vi "UHR-Fleezers Control (host) - 11.9c.vi"() -> ()   [LabVIEW 2014] (continued)
        n2850 = Multiply(x=w4184, y=u64 2) -> (x*y=w4169:u64)
        n2851 = call "integrate 1D array interval - double.vi"("Ave N"=w4186, "Array In"=w4185) -> ("Array Out"=w4197:dbl[])  [unwired: 1 out]
        n2852 = call "integrate 1D array interval - double.vi"("Ave N"=w4186, "Array In"=w4283) -> ("Array Out"=w4282:dbl[])  [unwired: 1 out]
        n2853 = Array Size(array=w4197) -> (size(s)=w4198:i32)
        n2854 = Array Size(array=w4282) -> (size(s)=w4284:i32)
        n2855 = Multiply(x=w4170, y=w4169) -> (x*y=w4200:u64)
        n2856 = Multiply(x=w4170, y=w4169) -> (x*y=w4292:u64)
        n2857 = call-poly <vilib>:"Mean.vi"("X"=w4232) -> ("mean"=w4216:dbl)  [unwired: 1 out]
        n2858 = Subtract(x=w4200, y=w4198) -> (x-y=w4191:u64)
        n2859 = call-poly <vilib>:"Mean.vi"("X"=w4234) -> ("mean"=w4221:dbl)  [unwired: 1 out]
        n2860 = call-poly <vilib>:"Mean.vi"("X"=w4233) -> ("mean"=w4219:dbl)  [unwired: 1 out]
        n2861 = call-poly <vilib>:"Mean.vi"("X"=w4197) -> ("mean"=w4188:dbl)  [unwired: 1 out]
        n2862 = Subtract(x=w4292, y=w4284) -> (x-y=w4226:u64)
        n2863 = call-poly <vilib>:"Mean.vi"("X"=w4282) -> ("mean"=w4223:dbl)  [unwired: 1 out]
        n2864 = Initialize Array(1.0 ("element"), w4191) -> (w4187:dbl[])
        n2865 = Initialize Array(1.0 ("element"), w4226) -> (w4217:dbl[])
        n2866 = Multiply(x=w4187, y=w4188) -> (x*y=w4189:dbl[])
        n2867 = Multiply(x=w4217, y=w4219) -> (x*y=w4220:dbl[])
        n2868 = Multiply(x=w4217, y=w4221) -> (x*y=w4222:dbl[])
        n2869 = Multiply(x=w4217, y=w4216) -> (x*y=w4218:dbl[])
        n2870 = Multiply(x=w4217, y=w4223) -> (x*y=w4224:dbl[])
        n2871 = Build Array (concatenate)(w4232, w4218) -> (w4286:dbl[])
        n2872 = Build Array (concatenate)(w4234, w4222) -> (w4290:dbl[])
        n2873 = Build Array (concatenate)(w4233, w4220) -> (w4289:dbl[])
        n2874 = Build Array (concatenate)(w4197, w4189) -> (w4199:dbl[])
        n2875 = Build Array (concatenate)(w4282, w4224) -> (w4291:dbl[])
        n2876 = Reshape Array(w4286, w4170, w4169) -> (w4252:dbl[][])
        n2877 = Reshape Array(w4199, w4170, w4169) -> (w4195:dbl[][])
        n2878 = Reshape Array(w4290, w4170, w4169) -> (w4244:dbl[][])
        n2879 = Reshape Array(w4289, w4170, w4169) -> (w4259:dbl[][])
        n2880 = Reshape Array(w4291, w4170, w4169) -> (w4269:dbl[][])
        n2881 = Array Subset(array=w4259, index (col)=0 ("index"), length (col)=w4184) -> (w4264:dbl[][])  [unwired: 2 in]
        n2882 = Array Subset(array=w4259, index (col)=w4184) -> (w4262:dbl[][])  [unwired: 3 in]
        n2883 = Array Subset(array=w4244, index (col)=0 ("index"), length (col)=w4184) -> (w4250:dbl[][])  [unwired: 2 in]
        n2884 = Array Subset(array=w4244, index (col)=w4184) -> (w4248:dbl[][])  [unwired: 3 in]
        n2885 = Array Subset(array=w4195, index (col)=0 ("index"), length (col)=w4184) -> (w4194:dbl[][])  [unwired: 2 in]
        n2886 = Array Subset(array=w4195, index (col)=w4184) -> (w4192:dbl[][])  [unwired: 3 in]
        n2887 = Array Subset(array=w4269, index (col)=0 ("index"), length (col)=w4184) -> (w4268:dbl[][])  [unwired: 2 in]
        n2888 = Array Subset(array=w4269, index (col)=w4184) -> (w4266:dbl[][])  [unwired: 3 in]
        n2889 = Array Subset(array=w4252, index (col)=0 ("index"), length (col)=w4184) -> (w4257:dbl[][])  [unwired: 2 in]
        n2890 = Array Subset(array=w4252, index (col)=w4184) -> (w4255:dbl[][])  [unwired: 3 in]
        n2891 = for {
          tunnel: w4264 -> [w4306] mode=indexing
          tunnel: [w4305] -> w4263 mode=indexing
          workers-P: _ -> [_]
          n2892 = Reverse 1D Array(array=w4306) -> (reversed array=w4305:dbl[])
        }
        n2893 = for {
          tunnel: w4250 -> [w4302] mode=indexing
          tunnel: [w4301] -> w4249 mode=indexing
          workers-P: _ -> [_]
          n2894 = Reverse 1D Array(array=w4302) -> (reversed array=w4301:dbl[])
        }
        n2895 = for {
          tunnel: w4194 -> [w4300] mode=indexing
          tunnel: [w4299] -> w4193 mode=indexing
          workers-P: _ -> [_]
          n2896 = Reverse 1D Array(array=w4300) -> (reversed array=w4299:dbl[])
        }
        n2897 = for {
          tunnel: w4268 -> [w4308] mode=indexing
          tunnel: [w4307] -> w4267 mode=indexing
          workers-P: _ -> [_]
          n2898 = Reverse 1D Array(array=w4308) -> (reversed array=w4307:dbl[])
        }
        n2899 = for {
          tunnel: w4257 -> [w4304] mode=indexing
          tunnel: [w4303] -> w4256 mode=indexing
          workers-P: _ -> [_]
          n2900 = Reverse 1D Array(array=w4304) -> (reversed array=w4303:dbl[])
        }
        n2901 = Index Array(array=w4269, index (row)=0) -> (element=→"Waveform Graph":dbl[])  [unwired: 1 in]
        n2902 = Add(x=w4263, y=w4262) -> (x+y=w4261:dbl[][])
        n2903 = Add(x=w4249, y=w4248) -> (x+y=w4247:dbl[][])
        n2904 = Add(x=w4193, y=w4192) -> (x+y=w4177:dbl[][])
        n2905 = Add(x=w4267, y=w4266) -> (x+y=w4241:dbl[][])
        n2906 = Add(x=w4256, y=w4255) -> (x+y=w4254:dbl[][])
        n2907 = Divide(x=w4247, y=2) -> (x/y=w4245:dbl[][])
        n2908 = Divide(x=w4261, y=2) -> (x/y=w4206:dbl[][])
        n2909 = Divide(x=w4254, y=2) -> (x/y=w4208:dbl[][])
        n2910 = To Single Precision Float(number=w4241) -> (single precision float=w4240:sgl[][])
        n2911 = Transpose 2D Array(2D array=w4245) -> (transposed array=→"Data map":dbl[][])
        n2912 = To Single Precision Float(number=w4177) -> (single precision float=w4181:sgl[][])
        n2913 = To Single Precision Float(number=w4206) -> (single precision float=w4212:sgl[][])
        n2914 = To Single Precision Float(number=w4208) -> (single precision float=w4209:sgl[][])
        n2915 = call "IMAQ ArrayToImage"("Image Pixels (Float)"=w4240, "Image"=w4174) -> ("Image Out"=w4243:T2)  [unwired: 8 in, 1 out]
        n2916 = call "IMAQ ArrayToImage"("Image Pixels (Float)"=w4181, "Image"=w4173) -> ("Image Out"=w4183:T2)  [unwired: 8 in, 1 out]
        n2917 = call "IMAQ ArrayToImage"("Image Pixels (Float)"=w4212, "Image"=w4172) -> ("Image Out"=w4214:T2)  [unwired: 8 in, 1 out]
        n2918 = call "IMAQ ArrayToImage"("Image Pixels (Float)"=w4209, "Image"=w4171) -> ("Image Out"=w4211:T2)  [unwired: 8 in, 1 out]
        n2919 = call "IMAQ Symmetry"("Type of Symmetry"=w4242, "Image Src"=w4243) -> ("Image Dst Out"=w4238:T2)  [unwired: 3 in, 1 out]
        n2920 = call "IMAQ Symmetry"("Type of Symmetry"=w4182, "Image Src"=w4183) -> ("Image Dst Out"=w4179:T2)  [unwired: 3 in, 1 out]
        n2921 = call "IMAQ Symmetry"("Type of Symmetry"=w4213, "Image Src"=w4214) -> ("Image Dst Out"=→"Detection Laser X":T2)  [unwired: 3 in, 1 out]
        n2922 = call "IMAQ Symmetry"("Type of Symmetry"=w4210, "Image Src"=w4211) -> ("Image Dst Out"=→"Detection Laser Y":T2)  [unwired: 3 in, 1 out]
        n2923 = call "IMAQ Set Simple Calibration"("Calibration Axis Info"=T37 {"Origin Pixel"={"X"=0.0, "Y"=0.0}, "Angle Relative to Horizontal (deg)"=0.0, "Axis Reference"=0}, "Grid Descriptor"=T38 {"X Step"=0.3, "Y Step"=0.3, "Unit"=enum."Undefined"}, "Image"=w4238) -> ("Calibrated Image"=→"APD 1":T2)  [unwired: 7 in, 1 out]
        n2924 = call "IMAQ Set Simple Calibration"("Calibration Axis Info"=T37 {"Origin Pixel"={"X"=0.0, "Y"=0.0}, "Angle Relative to Horizontal (deg)"=0.0, "Axis Reference"=0}, "Grid Descriptor"=T38 {"X Step"=0.3, "Y Step"=0.3, "Unit"=enum."Undefined"}, "Image"=w4179) -> ("Calibrated Image"=→"APD 2":T2)  [unwired: 7 in, 1 out]
      }
    }
    n2925 = Subtract(x=w3621, y="APD 2 Offset") -> (x-y=w3618:waveform(dbl))
    n2926 = Subtract(x=w3623, y="APD 1 Offset") -> (x-y=w3619:waveform(dbl))
    n2927 = Index Array(array=w3638, index=3) -> (element=w3698:waveform(dbl))
    n2928 = Index Array(array=w3638, index=6) -> (element=w3695:waveform(dbl))
    n2929 = Build Array(w3619, w3618) -> (→"APD Chart":waveform(dbl)[])
    n2930 = Array Size(array=w3689) -> (size(s)=w3742:i32)
    n2931 = call <vilib>:"Std Deviation and Variance.vi"("X"=w3631) -> ("standard deviation"=w3630:dbl)  [unwired: 1 in, 2 out]
    n2932 = Add Array Elements(numeric array=w3631) -> (sum=w3633:u32)
    n2933 = Add Array Elements(numeric array=w3689) -> (sum=w3752:u32)
    n2934 = call <vilib>:"Std Deviation and Variance.vi"("X"=w3689) -> ("standard deviation"=w3688:dbl)  [unwired: 1 in, 2 out]
    n2935 = Divide(x="T1 offset_x (mV)", y=1000.0) -> (x/y=w3699:dbl)
    n2936 = Divide(x=w3630, y=w3629) -> (x/y=w3626:dbl)
    "Rate sigma (Hz) 2" <- w3626
    n2937 = Multiply(x=w3629, y=w3742) -> (x*y=w3632:dbl)
    "Int. Time (s)" <- w3632
    n2938 = Divide(x=w3633, y=w3632) -> (x/y=w3627:dbl)
    "APD 2 Rate (Hz)" <- w3627
    n2939 = Divide(x=w3752, y=w3632) -> (x/y=w3686:dbl)
    "APD 1 Rate (Hz)" <- w3686
    n2940 = Divide(x=w3688, y=w3629) -> (x/y=w3687:dbl)
    "Rate sigma (Hz)" <- w3687
    n2941 = Divide(x=w3626, y=w3627) -> (x/y=→"Sigma/Mean 2":dbl)
    n2942 = Divide(x=w3687, y=w3686) -> (x/y=→"s/Mean":dbl)
    n2943 = feedback-in #26("Calibration") -> ()
    n2944 = feedback #26(u16 1 ("Calibration")) -> (w3719:u16)
    n2945 = Divide(x="T2 offset_x (mV)", y=1000.0) -> (x/y=w3697:dbl)
    n2946 = case shown="0, Default" "Calibration" {
      tunnel: "T1 a_x (nm/V)" -> [_ w4137 w4158]
      tunnel: "T1 k_x (pN/nm)" -> [_ _ w4148]
      tunnel: "T2 a_x (nm/V)" -> [_ w4136 w4156]
      tunnel: "T2 k_x (pN/nm)" -> [_ _ w4149]
      tunnel: w3698 -> [w4119 w4134 w4154]
      tunnel: w3695 -> [w4118 w4132 w4152]
      tunnel: [w4119 w4131 w4151] -> w3728
      tunnel: [w4118 w4130 w4150] -> w3727
      tunnel: ["T1 X (V)" ("Label.Text") "T1 X (nm)" ("Label.Text") "T1 X (pN)" ("Label.Text")] -> w3716
      tunnel: ["T2 X (V)" ("Label.Text") "T2 X (nm)" ("Label.Text") "T2 X (pN)" ("Label.Text")] -> w3715
      tunnel: ["Position (V)" ("Label.Text") "Position (nm)" ("Label.Text") "Force (pN)" ("Label.Text")] -> w3717
      tunnel: w3697 -> [_ w4122 w4141]
      tunnel: w3699 -> [_ w4125 w4143]
      tunnel: ["Mean (V)" ("Label.Text") "Mean (nm)" ("Label.Text") "Mean (pN)" ("Label.Text")] -> w3712
      tunnel: ["Difference (V)" ("Label.Text") "Difference (nm)" ("Label.Text") "Difference (pN)" ("Label.Text")] -> w3646
      frame 0, Default {
      }
      frame 1 {
        n2947 = Unbundle By Name(w4134) -> ("Y"=w4138:dbl[])
        n2948 = Unbundle By Name(w4132) -> ("Y"=w4123:dbl[])
        n2949 = Subtract(x=w4138, y=w4125) -> (x-y=w4126:dbl[])
        n2950 = Subtract(x=w4123, y=w4122) -> (x-y=w4124:dbl[])
        n2951 = Multiply(x=w4124, y=w4136) -> (x*y=w4133:dbl[])
        n2952 = Multiply(x=w4137, y=w4126) -> (x*y=w4135:dbl[])
        n2953 = Bundle By Name(cluster=w4132, "Y"=w4133) -> (w4130:waveform(dbl))
        n2954 = Bundle By Name(cluster=w4134, "Y"=w4135) -> (w4131:waveform(dbl))
      }
      frame 2 {
        n2955 = Unbundle By Name(w4154) -> ("Y"=w4159:dbl[])
        n2956 = Unbundle By Name(w4152) -> ("Y"=w4157:dbl[])
        n2957 = Subtract(x=w4157, y=w4141) -> (x-y=w4142:dbl[])
        n2958 = Subtract(x=w4159, y=w4143) -> (x-y=w4144:dbl[])
        n2959 = Compound Arithmetic op=MULTIPLY(w4142, w4156, w4149) -> (w4153:dbl[])
        n2960 = Compound Arithmetic op=MULTIPLY(w4148, w4158, w4144) -> (w4155:dbl[])
        n2961 = Bundle By Name(cluster=w4152, "Y"=w4153) -> (w4150:waveform(dbl))
        n2962 = Bundle By Name(cluster=w4154, "Y"=w4155) -> (w4151:waveform(dbl))
      }
    }
    n2963 = Not Equal?(x=w3719, y="Calibration") -> (x != y?=w3676:bool)
    n2964 = case shown="True" w3676 {
      tunnel: w3717 -> [_ w4112]
      tunnel: w3716 -> [_ w4111]
      tunnel: w3715 -> [_ w4110]
      tunnel: w3712 -> [_ w4109]
      tunnel: w3646 -> [_ w4108]
      frame False {
      }
      frame True {
        n2965 = property on="Force" class="WFChart (strict)"("YScale.NameLbl.Text"=w4112) -> ()  [unwired: 2 in, 2 out]
        n2966 = property on="T2 X" class="DigNum (strict)"("Caption.Text"=w4110) -> ()  [unwired: 2 in, 2 out]
        n2967 = property on="T1 X" class="DigNum (strict)"("Caption.Text"=w4111) -> ()  [unwired: 2 in, 2 out]
        n2968 = property on="Mean" class="DigNum (strict)"("Caption.Text"=w4109) -> ()  [unwired: 2 in, 2 out]
        n2969 = property on="Difference" class="DigNum (strict)"("Caption.Text"=w4108) -> ()  [unwired: 2 in, 2 out]
      }
    }
    n2970 = Unbundle By Name(w3698) -> ("Y"=w3701:dbl[])
    n2971 = Unbundle By Name(w3695) -> ("Y"=w3704:dbl[])
    n2972 = Subtract(x=w3701, y=w3699) -> (x-y=w3702:dbl[])
    n2973 = Subtract(x=w3704, y=w3697) -> (x-y=w3703:dbl[])
    n2974 = Multiply(x=w3703, y="T2 a_x (nm/V)") -> (x*y=w3491:dbl[])
    n2975 = Multiply(x="T1 a_x (nm/V)", y=w3702) -> (x*y=w3492:dbl[])
    n2976 = Not(x="Trap Trig. Fl.") -> (.not. x?=w3528:bool)
    n2977 = Multiply(x=w3727, y=-1.0) -> (x*y=w3706:waveform(dbl))
    n2978 = Subtract(x=w3492, y=w3491) -> (x-y=w3694:dbl[])
    n2979 = Unbundle By Name(w3727) -> ("Y"=w3665:dbl[])
    n2980 = Unbundle By Name(w3728) -> ("Y"=w3493:dbl[])
    n2981 = Negate(x=w3694) -> (-x=w3489:dbl[])
    n2982 = Build Array(w3728, w3706) -> (→"Force":waveform(dbl)[])
    n2983 = Subtract(x=w3489, y="Offset (nm)") -> (x-y=w3663:dbl[])
    n2984 = case shown="True" "Read Lateness and Rel Phase" {
      tunnel: w3509 -> [w4083 w4107]
      tunnel: w3508 -> [w4084 w4106]
      tunnel: [w4083 w4105] -> w3692
      tunnel: [w4084 w4104] -> w3691
      frame False {
      }
      frame True {
        n2985 = xnode "Read/Write Control"("FPGA VI Reference In"=w4107, "error in"=w4106) -> ("FPGA VI Reference Out"=w4105:T20, "error out"=w4104:errorcluster, "GI Relative phase"=→"GI relative phase":i16, "Relative phase"=→"Relative phase (AI1)":i16, "AI Late Counter"=→"Late Counter (AI1)":u8, "GI Late Counter"=→"GI Late Counter":u8, "MCL Late Counter"=→"MCL Late Counter":u8, "MCL Relative Phase"=→"Relative Phase (MCL)":i16, "APD Acq Relative Phase"=→"APD Acq Relative Phase":i16, "APD 1 Gate Relative Phase"=→"APD 1 Gate Relative Phase":i16, "APD 2 Gate Relative Phase"=→"APD 2 Gate Relative Phase":i16, "APD Acq Late Counter"=→"APD Acq Late Counter":u8, "APD 1 Gate Late Counter"=→"APD 1 Gate Late Counter":u8, "APD 2 Gate Late Counter"=→"APD 2 Gate Late Counter":u8, "Green FB Relative Phase"=→"Relative phase (Green FB)":i16, "GI Relative phase 2"=→"GI relative phase 2":i16, "GI Late Counter 2"=→"GI Late Counter 2":u8, "Trap Pos FIFO Timeout"=→"Trap Pos FIFO Timeout":u16, "Trap AI FIFO Timeout"=→"Trap AI FIFO Timeout":u16, "RI relative phase"=→"RI relative phase":i16, "RI late counter"=→"RI late counter":u8)
      }
    }
    n2986 = call-poly <vilib>:"Mean.vi"("X"=w3665) -> ("mean"=w3495:dbl)  [unwired: 1 out]
    "T2 X" <- w3495
    n2987 = Negate(x=w3665) -> (-x=w3666:dbl[])
    n2988 = call-poly <vilib>:"Mean.vi"("X"=w3493) -> ("mean"=w3496:dbl)  [unwired: 1 out]
    "T1 X" <- w3496
    n2989 = Negate(x=w3495) -> (-x=w3494:dbl)
    n2990 = Bundle By Name(cluster=w3698, "Y"=w3663) -> (w3637:waveform(dbl))
    "Bead Separation" <- w3637
    n2991 = Add(x=w3493, y=w3666) -> (x+y=w3667:dbl[])
    n2992 = Add(x=w3496, y=w3494) -> (x+y=w3714:dbl)
    n2993 = Subtract(x=w3496, y=w3494) -> (x-y=→"Difference":dbl)
    n2994 = Divide(x=w3667, y=2.0) -> (x/y=→"Vec Mean of T1 T2":dbl[])
    n2995 = Divide(x=w3714, y=2.0) -> (x/y=w3669:dbl)
    "Mean" <- w3669
    n2996 = feedback-in #27("Trap Trig. Fl.") -> ()
    n2997 = feedback #27("Trap Trig. Fl.") -> (w3526:bool)
    n2998 = And(x=w3528, y=w3526) -> (x .and. y?=w3527:bool)
    n2999 = case "If have just turned off triggering" shown="True" w3527 {
      tunnel: w3509 -> [_ w3913]
      tunnel: w3508 -> [_ w3912]
      frame False {
      }
      frame True {
        w3911 = FALSE ("FPGA Trap Trig")
        n3000 = xnode "Read/Write Control"("FPGA VI Reference In"=w3913, "error in"=w3912, "FPGA Trap Trig"=w3911) -> ("FPGA VI Reference Out"=w3910:T20, "error out"=w3909:errorcluster)
        n3001 = xnode "Read/Write Control"("FPGA VI Reference In"=w3910, "error in"=w3909, "TTrig?"=w3911) -> ()  [unwired: 2 out]
        n3002 = local write "Initializing"(FALSE ("Initializing")) -> ()
        n3003 = local write "Triggered"(FALSE ("Triggered")) -> ()
        n3004 = local write "Waiting"(FALSE ("Waiting")) -> ()
      }
    }
    n3005 = Not(x=w3526) -> (.not. x?=w3539:bool)
    n3006 = And(x="Trap Trig. Fl.", y=w3539) -> (x .and. y?=w3536:bool)
    n3007 = local read "Tether"() -> (w3670:bool)
    n3008 = Or(x=w3536, y="Reinitialize") -> (x .or. y?=w3522:bool)
    n3009 = feedback #28(w3532) -> (w3537:string)
    n3010 = Select(t=w3532, s=w3536, f=w3537) -> (s? t:f=w3531:string)
    n3011 = Select(t=w3532, s="Reinitialize", f=w3531) -> (s? t:f=w3530:string)
    n3012 = feedback #29(0) -> (w3534:i32)
    n3013 = feedback #30(w3663) -> (w3662:dbl[])
    n3014 = Build Array (concatenate)(w3663, w3662) -> (w3490:dbl[])
    n3015 = case "For determining if there is a tether still" shown="True" w3670 {
      tunnel: w3669 -> [_ w4037]
      frame False {
      }
      frame True {
        n3016 = Greater?(x="Lost Tether Alarm Threshold (pN)", y=w4037) -> (0:w4035:bool)
        n3017 = case shown="True" w4035 {
          frame False {
          }
          frame True {
            w4038 = TRUE
            w4042 = FALSE ("Multiple tether")
            w4043 = FALSE ("Value (Signaling)")
            n3018 = flat-sequence {
              frame #0 {
                # "stop only if saving"
                n3019 = local read "Saving..."() -> (w4055:bool)
                n3020 = And(x=w4055, y="TA Cancel Save?") -> (x .and. y?=w4054:bool)
                n3021 = local write "Stop Saving"(w4054) -> ()
              }
              frame #1 {
                n3022 = case shown="True" "TA Green Off?" {
                  frame False {
                  }
                  frame True {
                    w4058 = FALSE ("Fl. Triggered...")
                    n3023 = local write "Fl. Triggered..."(w4058) -> ()
                    n3024 = property on="Green ON/Interlacing" class="Bool (strict)"("Val(Sgnl)"=w4058) -> ()  [unwired: 2 in, 2 out]
                  }
                }
              }
            }
            n3025 = local read "Time tether formed"() -> (w4049:timestamp)
            n3026 = Get Date/Time In Seconds() -> (seconds since 1Jan1904=w4050:timestamp)
            n3027 = Subtract(x=w4050, y=w4049) -> (x-y=w4048:dbl)
            n3028 = Number To Decimal String(number=w4048) -> (decimal integer string=w4045:string)  [unwired: 1 out]
            n3029 = local read "Messages"() -> (w4052:string)
            n3030 = call <vilib>:"Beep.vi"("use system alert? (T)"=FALSE, "duration (msec)"=u32 200, "frequency (Hz)"=u32 200) -> ()  [unwired: 9 out]
            n3031 = Concatenate Strings("Lost tether (" ("Message to add"), w4045, " s)." ("string")) -> (w4047:string)
            n3032 = local write "Tether"(FALSE ("Tether")) -> ()
            n3033 = call "Update messages.vi"("Message to add"=w4047, "Old message string"=w4052) -> ("New message string"=w4051:string)
            n3034 = local write "Messages"(w4051) -> ()
            n3035 = local write "Pause dwell"(w4043) -> ()
            n3036 = property on="Fl. Triggered..." class="Bool (strict)"("Val(Sgnl)"=w4043) -> ()  [unwired: 2 in, 2 out]
            n3037 = local write "Dip for Protein"(w4043) -> ()
            n3038 = property on="Trap Pos. FB ON" class="Bool (strict)"("Val(Sgnl)"=w4043) -> ()  [unwired: 2 in, 2 out]
            n3039 = property on="Trap Trig. Fl." class="Bool (strict)"("Val(Sgnl)"=w4043) -> ()  [unwired: 2 in, 2 out]
            n3040 = local write "Multiple tether"(w4042) -> ()
            n3041 = local write "Bad fit"(w4042) -> ()
            n3042 = local write "Hysteresis"(w4042) -> ()
            n3043 = local write "Good tether"(w4042) -> ()
            n3044 = local write "Save scans"(w4038) -> ()
            n3045 = local write "Restart DMA? (AOD)"(w4038) -> ()
          }
        }
      }
    }
    n3046 = case "For triggering actions based on the trap position (e.g., turning the excitation laser on if trap under feedback moves so far)" shown="True" "Trap Trig. Fl." {
      tunnel: w3517 -> [_ w3926]
      tunnel: w3530 -> [_ w3925]
      tunnel: ["" ("t") w3924] -> w3538
      tunnel: w3522 -> [_ w3923]
      tunnel: [0 ("t") w3922] -> w3535
      tunnel: w3534 -> [_ w3921]
      tunnel: w3509 -> [_ w3920]
      tunnel: w3508 -> [_ w3919]
      frame False {
      }
      frame True {
        n3047 = case shown="\"Wait for trigger\"" w3925 {
          tunnel: w3926 -> [w3943 _ _ w3991]
          tunnel: [w3940 w3972 "" ("t") w3994] -> w3924
          tunnel: w3923 -> [_ _ _ w3982]
          tunnel: [w3939 w3969 0 ("t") w3983] -> w3922
          tunnel: w3921 -> [_ w3971 _ w3989]
          tunnel: w3920 -> [w3928 w3966 _ w3985]
          tunnel: w3919 -> [w3927 w3965 _ w3984]
          frame "Wait for trigger" {
            n3048 = local read "Trap Trig. (FPGA)"() -> (w3931:bool)
            n3049 = Subtract(x=w3943, y="Mean T1 Position\nto compare (nm)") -> (x-y=w3936:dbl[])
            n3050 = call <vilib>:"Std Deviation and Variance.vi"("X"=w3936) -> ("mean"=→"mean":dbl, "standard deviation"=→"standard\ndeviation":dbl)  [unwired: 1 in, 1 out]
            n3051 = Array Max & Min(array=w3936) -> (max value=→"max value":dbl, min value=→"min value":dbl)  [unwired: 2 out]
            n3052 = Greater?(x=w3936, y="Threshold (nm)") -> (0:w3946:bool[])
            n3053 = case shown="True" w3931 {
              tunnel: w3928 -> [_ w3952]
              tunnel: w3927 -> [_ w3951]
              tunnel: [FALSE ("TTrig?") w3950] -> w3934
              frame False {
              }
              frame True {
                n3054 = xnode "Read/Write Control"("FPGA VI Reference In"=w3952, "error in"=w3951) -> ("TTrig?"=w3950:bool)  [unwired: 2 out]
              }
            }
            n3055 = Or Array Elements(Boolean array=w3946) -> (logical OR=w3933:bool)
            n3056 = Select(t=w3934, s=w3931, f=w3933) -> (s? t:f=w3932:bool)
            n3057 = Not(x=w3931) -> (.not. x?=w3930:bool)
            n3058 = And(x=w3932, y=w3930) -> (x .and. y?=w3929:bool)
            n3059 = Select(t="Triggered", s=w3932, f="Wait for trigger") -> (s? t:f=w3940:string)
            n3060 = case shown="True" w3932 {
              tunnel: [0 0] -> w3939
              tunnel: w3928 -> [_ w3957]
              tunnel: w3927 -> [_ w3956]
              frame False {
                "Waiting" <- TRUE ("Waiting")
              }
              frame True {
                n3061 = xnode "Read/Write Control"("FPGA VI Reference In"=w3957, "error in"=w3956, "TTrig?"=FALSE) -> ()  [unwired: 2 out]
                n3062 = local read "Messages"() -> (w3960:string)
                n3063 = call <vilib>:"Beep.vi"() -> ()  [unwired: 12 in]
                n3064 = call "Update messages.vi"("Message to add"="Unwinding trigger.", "Old message string"=w3960) -> ("New message string"=w3961:string)
                n3065 = local write "Messages"(w3961) -> ()
                n3066 = local write "Waiting"(FALSE ("Waiting")) -> ()
                "Triggered" <- TRUE ("Triggered")
              }
            }
            n3067 = case "Only need to turn on laser if host triggered" shown="True" w3929 {
              frame False {
              }
              frame True {
                n3068 = property on="Green ON/Interlacing" class="Bool (strict)"("Val(Sgnl)"=TRUE ("Value (Signaling)")) -> ()  [unwired: 2 in, 2 out]
              }
            }
          }
          frame "Triggered" {
            n3069 = local read "Trap Trig. (FPGA)"() -> (w3968:bool)
            n3070 = Increment(x=w3971) -> (x+1=w3969:i32)
            n3071 = Greater Or Equal?(x=w3969, y="Fl. ON time (n)") -> (x >= y?=w3967:bool)
            n3072 = Select(t="Wait for trigger", s=w3967, f="Triggered" ("t")) -> (s? t:f=w3972:string)
            n3073 = And(x=w3967, y=w3968) -> (x .and. y?=w3964:bool)
            n3074 = case shown="True" w3964 {
              tunnel: w3966 -> [_ w3976]
              tunnel: w3965 -> [_ w3975]
              frame False {
              }
              frame True {
                n3075 = xnode "Read/Write Control"("FPGA VI Reference In"=w3976, "error in"=w3975, "FPGA Trap Trig"=TRUE) -> ()  [unwired: 2 out]
              }
            }
            n3076 = case shown="True" w3967 {
              frame False {
              }
              frame True {
                w3978 = FALSE ("Value (Signaling)")
                n3077 = local write "Triggered"(w3978) -> ()
                n3078 = local write "Waiting"(TRUE ("Waiting")) -> ()
                n3079 = property on="Green ON/Interlacing" class="Bool (strict)"("Val(Sgnl)"=w3978) -> ()  [unwired: 2 in, 2 out]
              }
            }
          }
          frame "Do nothing" {
          }
          frame "Initialize", Default {
            n3080 = Increment(x=w3989) -> (x+1=w3993:i32)
            n3081 = Select(t=1, s=w3982, f=w3993) -> (s? t:f=w3983:i32)
            n3082 = feedback #31(w3991) -> (w3997:dbl[])
            n3083 = Build Array (concatenate)(w3991, w3997) -> (w3990:dbl[])
            n3084 = Greater Or Equal?(x=w3983, y="Wait to get offset (n)") -> (x >= y?=w3986:bool)
            n3085 = Select(t=w3991, s=w3982, f=w3990) -> (s? t:f=w3992:dbl[])
            n3086 = feedback-in #31(w3992) -> ()
            n3087 = call-poly <vilib>:"Mean.vi"("X"=w3992) -> ("mean"=w3987:dbl)  [unwired: 1 out]
            n3088 = local write "Mean T1 Position\nto compare (nm)"(w3987) -> ()
            n3089 = case shown="True" w3982 {
              tunnel: w3985 -> [_ w4003]
              tunnel: w3984 -> [_ w4002]
              frame False {
              }
              frame True {
                w3999 = FALSE ("FPGA Trap Trig")
                n3090 = xnode "Read/Write Control"("FPGA VI Reference In"=w4003, "error in"=w4002, "FPGA Trap Trig"=w3999) -> ("FPGA VI Reference Out"=w4001:T20, "error out"=w4000:errorcluster)
                n3091 = xnode "Read/Write Control"("FPGA VI Reference In"=w4001, "error in"=w4000, "TTrig?"=w3999) -> ()  [unwired: 2 out]
              }
            }
            n3092 = Select(t="Wait for trigger", s=w3986, f="Initialize") -> (s? t:f=w3994:string)
            n3093 = case shown="True" w3986 {
              tunnel: w3987 -> [_ w4006]
              tunnel: w3985 -> [_ w4015]
              tunnel: w3984 -> [_ w4014]
              frame False {
                n3094 = local write "Waiting"(FALSE ("Waiting")) -> ()
                "Initializing" <- TRUE ("Initializing")
              }
              frame True {
                n3095 = local read "Threshold (nm)"() -> (w4018:dbl)
                n3096 = local read "AOM X Cal (nm/MHz)"() -> (w4017:dbl)
                n3097 = Add(x=w4006, y=w4018) -> (x+y=w4019:dbl)
                n3098 = Divide(x=w4019, y=w4017) -> (x/y=w4016:dbl)
                n3099 = call "IR AOM freq to word.vi"("Frequency In (MHz)"=w4016) -> ("Frequency Word Out (double)"=w4013:dbl)
                n3100 = local write "Initializing"(FALSE ("Initializing")) -> ()
                n3101 = local write "Waiting"(TRUE ("Waiting")) -> ()
                n3102 = To Quad Integer(1:w4013) -> (0:w4012:i64)
                n3103 = xnode "Read/Write Control"("FPGA VI Reference In"=w4015, "error in"=w4014, "FPGA TTrig Thresh"=w4012) -> ("FPGA VI Reference Out"=w4009:T20, "error out"=w4008:errorcluster)
                n3104 = xnode "Read/Write Control"("FPGA VI Reference In"=w4009, "error in"=w4008, "FPGA Trap Trig"=TRUE) -> ()  [unwired: 2 out]
              }
            }
          }
        }
      }
    }
    n3105 = feedback-in #28(w3538) -> ()
    n3106 = feedback-in #29(w3535) -> ()
    n3107 = Split 1D Array(array=w3490, index=w3552) -> (first subarray=w3659:dbl[])  [unwired: 1 out]
    n3108 = feedback-in #30(w3659) -> ()
    n3109 = call-poly <vilib>:"Mean.vi"("X"=w3659) -> ("mean"=w3658:dbl)  [unwired: 1 out]
    "Bead Mean (nm)" <- w3658
    n3110 = Subtract(x=w3659, y=w3658) -> (x-y=w3657:dbl[])
    n3111 = Square(x=w3657) -> (x^2=w3656:dbl[])
    n3112 = call-poly <vilib>:"Mean.vi"("X"=w3656) -> ("mean"=w3655:dbl)  [unwired: 1 out]
    n3113 = Square Root(x=w3655) -> (sqrt(x)=w3654:dbl)
    n3114 = Multiply(x=10.0, y=w3654) -> (x*y=→"RMS (Å)":dbl)
    n3115 = xnode ("Read/Write Control")("FPGA VI Reference In"=w3692, "error in"=w3691) -> ("FPGA VI Reference Out"=w3520:T20, "error out"=w3519:errorcluster, "AI2 Y Sum Set 1"=w3796:i16, "AI2 Y Sum Set 2"=w3795:i16, "AI1 X Set 1"=w3583:fxp<+/-,16,1>, "AI1 X Set 2"=w3582:fxp<+/-,16,1>, "Trap Pos FB Int Signal"=→"Trap Pos FB Int Signal":fxp<+/-,24,9>, "Trap Pos FB Int-Norm Signal"=→"Trap Pos FB Int-Norm Signal":fxp<+/-,16,1>, "Trap Pos FB Action"=w3576:i64, "Scanning"=→"AOD Scanning":bool, "Scan I"=→"AOD Scan I":u64, "Scanning MCL"=w3798:bool, "Scan I (MCL)"=→"MCL Scan I":u64, "Green FB Signals"=w3737:T48, "Trap Pos FB Action"=w3507:i64, "Wiggling 1"=→"Wiggling T1":bool, "TTrig Fin Thresh"=w3503:i64, "Wiggling 2"=→"Wiggling T2":bool)  [unwired: 2 out]
    "MCL Scanning" <- w3798
    "Trap Pos FB Action" <- w3576
    n3116 = local read "FB Trig Integrate"() -> (w3501:u32)
    n3117 = Divide(x=w3507, y=w3501) -> (x/y=w3500:dbl)
    "TTrig Sig (Int)" <- w3500
    n3118 = Divide(x=w3503, y=w3501) -> (x/y=w3498:dbl)
    "TTrig Fin Thresh (Int)" <- w3498
    n3119 = local read "AOM X Cal (nm/MHz)"() -> (w3506:dbl)
    n3120 = local read "AI2 (V)"() -> (w3797:cluster{"Set 1":dbl, "Set 2":dbl})
    n3121 = Bundle By Name(cluster=w3797, "Set 1"=w3796, "Set 2"=w3795) -> (w3793:cluster{"Set 1":dbl, "Set 2":dbl})
    n3122 = Divide(x=w3576, y=327.67) -> (x/y=w3485:dbl)
    n3123 = local read "Trap X (AI1)"() -> (w3596:T10)
    n3124 = call "IR AOM word double to freq.vi"("Frequency Word In (double)"=w3498) -> ("Frequency Out (MHz)"=w3497:dbl)
    n3125 = call "IR AOM word double to freq.vi"("Frequency Word In (double)"=w3500) -> ("Frequency Out (MHz)"=w3499:dbl)
    n3126 = Divide(x=w3793, y=3276.7) -> (x/y=w3792:cluster{"Set 1":dbl, "Set 2":dbl})
    n3127 = Multiply(x=w3499, y=w3506) -> (x*y=w3505:dbl)
    "TTrig Sig (nm)" <- w3505
    n3128 = Multiply(x=w3497, y=w3506) -> (x*y=w3504:dbl)
    "TTrig Fin Thresh (nm)" <- w3504
    n3129 = local write "AI2 (V)"(w3792) -> ()
    n3130 = local read "Trap Pos. FB Range"() -> (w3484:T12)
    n3131 = Bundle(cluster=w3596, "Trap 1"=w3583, "Trap 2"=w3582) -> (→"Trap X (AI1)":T10)
    n3132 = Bundle(w3505, w3504) -> (→"TTrig":cluster{dbl, dbl})  [unwired: 1 in]
    n3133 = Unbundle(w3484) -> ("output high"=w3483:fxp<+/-,64,32>)  [unwired: 1 out]
    n3134 = Divide(x=w3485, y=w3483) -> (x/y=→"Action (%)":dbl)
    n3135 = Divide(x=w3737, y=3276.7) -> (x/y=w3733:T49)
    n3136 = Unbundle By Name(w3733) -> ("Green FB Ch 0"=w3736:dbl, "Green FB Ch 1"=w3735:dbl, "Green FB Ch 2"=w3734:dbl)
    n3137 = Divide(x=w3736, y=w3734) -> (x/y=w3732:dbl)
    n3138 = Divide(x=w3735, y=w3734) -> (x/y=w3731:dbl)
    n3139 = flat-sequence "To save data" {
      tunnel: [w4881] -> w3816
      tunnel: [w4882] -> w3815
      tunnel: w3768 -> [w4854]
      tunnel: w3525 -> [w4879]
      tunnel: ["Save Calibration"] -> w3789
      tunnel: w3786 -> [w4878]
      tunnel: [w4872] -> w3785
      tunnel: [w4869] -> w3784
      tunnel: [w4866] -> w3783
      tunnel: w3767 -> [w4868]
      tunnel: w3674 -> [w4862]
      tunnel: [w4862] -> w3673
      tunnel: ["Start Saving"] -> w3639
      tunnel: [w4856] -> w3565
      tunnel: [w4855] -> w3564
      tunnel: w3816 -> [w5121]
      tunnel: w3815 -> [w5120]
      tunnel: w3566 -> [w5119]
      tunnel: w3789 -> [w5118]
      tunnel: w3785 -> [w5116]
      tunnel: w3784 -> [w5115]
      tunnel: w3783 -> [w5114]
      tunnel: w3648 -> [w5113]
      tunnel: w3684 -> [w5112]
      tunnel: w3673 -> [w5111]
      tunnel: w3639 -> [w5110]
      tunnel: w3637 -> [w5109]
      tunnel: w3613 -> [w5108]
      tunnel: w3565 -> [w5107]
      tunnel: w3564 -> [w5106]
      tunnel: w3563 -> [w5105]
      tunnel: w3486 -> [w5104]
      frame #0 {
        n3140 = Or(x="Save N Sets", y="Start Saving") -> (x .or. y?=w4863:bool)
        n3141 = To Double Precision Float(number=w4878) -> (double precision float=w4873:dbl)
        n3142 = Build Array(w4863, "Save Calibration", w4854, w4868) -> (w4877:bool[])
        n3143 = Compound Arithmetic op=OR("Save Calibration", w4854, w4863, w4868) -> (w4880:bool)
        n3144 = Boolean Array To Number(Boolean array=w4877) -> (number=w4875:u32)
        n3145 = feedback #32(FALSE ("Save APD Data\nwith Trap Data")) -> (w4857:bool)
        n3146 = feedback #33(refnum<k0> refnum) -> (w4883:refnum<file>)
        n3147 = feedback #34(refnum<k0> refnum) -> (w4859:refnum<file>)
        n3148 = feedback #35(FALSE ("Save APD Data\nwith Trap Data")) -> (w4867:bool)
        n3149 = feedback #36(refnum<k0> refnum) -> (w4870:refnum<file>)
        n3150 = feedback #37(0) -> (w4885:i32)
        n3151 = feedback #38() -> (w4874:u32)  [unwired: 1 out]
        n3152 = case shown="True" w4880 {
          tunnel: [w4892 1] -> w4881
          tunnel: w4885 -> [w4894 _]
          tunnel: [w4893 w4912] -> w4882
          tunnel: w4883 -> [w4893 _]
          tunnel: w4879 -> [_ w4932]
          tunnel: w4873 -> [_ w4930]
          tunnel: w4875 -> [_ w4933]
          tunnel: [w4891 w4911] -> w4872
          tunnel: w4874 -> [w4891 _]
          tunnel: [w4890 w4909] -> w4869
          tunnel: w4870 -> [w4890 _]
          tunnel: [w4889 w4908] -> w4866
          tunnel: w4867 -> [w4889 _]
          tunnel: "Start Saving" -> [_ w4906]
          tunnel: w4862 -> [_ w4905]
          tunnel: [w4888 w4896] -> w4855
          tunnel: w4859 -> [w4888 _]
          tunnel: [w4887 w4895] -> w4856
          tunnel: w4857 -> [w4887 _]
          frame False {
            n3153 = Increment(x=w4894) -> (x+1=w4892:i32)
          }
          frame True {
            w4902 = FALSE ("Start Saving")
            w4907 = 9.0  # File Version
            w4915 = FALSE ("prepend array or string size? (T)")
            w4913 = T25."big-endian, network order" ("byte order (0:big-endian, network order)")
            n3154 = local read "BD 1 Frequency 1 (MHz)"() -> (w4929:dbl)
            n3155 = local read "BD 2 Frequency 1 (MHz)"() -> (w4928:dbl)
            n3156 = local read "BD 1 Frequency 2 (MHz)"() -> (w4927:dbl)
            n3157 = local read "BD 2 Frequency 2 (MHz)"() -> (w4926:dbl)
            n3158 = local read "BD 1 Frequency 3 (MHz)"() -> (w4925:dbl)
            n3159 = local read "BD 2 Frequency 3 (MHz)"() -> (w4924:dbl)
            n3160 = Array Size(array=w4905) -> (size(s)=w4904:i32)
            n3161 = To Double Precision Float(number=w4904) -> (double precision float=w4903:dbl)
            n3162 = local write "Save Calibration"(w4902) -> ()
            n3163 = local write "Start Saving"(w4902) -> ()
            n3164 = Build Array("Save APD Data\nwith Trap Data", "Save Trap Pos. Data") -> (w4899:bool[])
            n3165 = Boolean Array To Number(Boolean array=w4899) -> (number=w4898:u32)
            n3166 = Build Array(w4929, w4928, w4927, w4926, w4925, w4924) -> (w4923:dbl[])
            n3167 = case shown="1, Default" w4933 {
              tunnel: w4932 -> [w5006 w5028 w5044 w5082]
              tunnel: w4903 -> [w5011 w5035 w5064 w5101]
              tunnel: w4930 -> [w5010 w5034 w5063 w5100]
              tunnel: [w5007 w5030 w5055 w5092] -> w4921
              tunnel: [w4999 "Cal sets to save" w5045 w5083] -> w4911
              tunnel: w4923 -> [w5008 w5031 w5057 w5094]
              tunnel: "Save APD Data\nwith Trap Data" -> [w5005 _ w5041 w5080]
              tunnel: [w5005 FALSE ("Save APD Data\nwith Trap Data") w5041 w5080] -> w4908
              tunnel: w4907 -> [w5002 w5025 w5039 w5078]
              tunnel: w4906 -> [w5001 _ _ _]
              tunnel: [w4993 "Active cal?" w5038 w5068] -> w4895
              tunnel: "Save Trap Pos. Data" -> [w4993 _ w5038 w5068]
              tunnel: w4898 -> [w4992 _ w5037 w5067]
              frame 1, Default {
                # "timeseries"
                n3168 = case shown="True" "Profile" {
                  tunnel: [w5014 w5018] -> w4997
                  tunnel: [w5014 w5017] -> w4996
                  tunnel: [w5014 w5016] -> w4995
                  tunnel: [w5014 w5015] -> w4994
                  frame False {
                    w5014 = 0.0 ("f")
                  }
                  frame True {
                    n3169 = local read "Current Position"() -> (w5019:cluster{dbl, dbl, dbl})
                    n3170 = local read "Y change (mm)"() -> (w5015:dbl)
                    n3171 = Unbundle(w5019) -> (w5018:dbl, w5017:dbl, w5016:dbl)
                  }
                }
                n3172 = local read "Save ave N"() -> (w5013:dbl)
                n3173 = Multiply(x=w5013, y=w5006) -> (x*y=w5012:dbl)
                n3174 = To Double Precision Float(number=w4992) -> (double precision float=w5004:dbl)
                n3175 = Select(t=4.0, s="Profile", f=0.0) -> (s? t:f=w4988:dbl)
                n3176 = Build Array(w5002, w5006, w5012, w5011, w5010, w4988) -> (w5009:dbl[])
                n3177 = Build Array(w5004, w4997, w4996, w4995, w4994) -> (w5003:dbl[])
                n3178 = Select(t=u32 4000000000, s=w5001, f="N sets to save") -> (s? t:f=w4999:u32)
                n3179 = Build Array (concatenate)(w5009, w5008, w5003) -> (w5007:dbl[])
              }
              frame 2 {
                w5027 = 0.0 ("f")
                # "If doing active calibration,\nalso save trap position file"
                # "calibration"
                n3180 = property on="Wiggle" class="Bool (strict)"("Val(Sgnl)"="Active cal?") -> ()  [unwired: 2 in, 2 out]
                n3181 = Select(t=2.0, s="Active cal?", f=0.0) -> (s? t:f=w5021:dbl)
                n3182 = Build Array(w5021, w5027, w5027, w5027, w5027) -> (w5026:dbl[])
                n3183 = Build Array(w5025, w5028, w5028, w5035, w5034, 1.0 ("t")) -> (w5032:dbl[])
                n3184 = Build Array (concatenate)(w5032, w5031, w5026) -> (w5030:dbl[])
                "Calibrating..." <- TRUE ("Calibrating...")
              }
              frame 4 {
                w5042 = 0.0 ("f")
                # "scan dir (x/y = 0/1)"
                # "cycles/step"
                # "n scans (f/b)"
                # "steps"
                # "freq. range"
                # "AOD raster scan"
                n3185 = local read "Number of F/B Scans (AOD)"() -> (w5049:u16)
                n3186 = local read "Cycles/step (AOD)"() -> (w5051:u64)
                n3187 = local read "Scan Range (MHz)"() -> (w5054:dbl)
                n3188 = local read "Scan steps (AOD)"() -> (w5053:u64)
                n3189 = local read "Scan BD"() -> (w5061:bool)
                n3190 = local read "Save ave N"() -> (w5066:dbl)
                n3191 = Boolean To (0,1)(Boolean=w5061) -> (0, 1=w5060:i16)
                n3192 = To Double Precision Float(number=w5049) -> (double precision float=w5048:dbl)
                n3193 = To Double Precision Float(number=w5053) -> (double precision float=w5052:dbl)
                n3194 = To Double Precision Float(number=w5051) -> (double precision float=w5050:dbl)
                n3195 = To Double Precision Float(number=w5060) -> (double precision float=w5059:dbl)
                n3196 = Multiply(x=w5066, y=w5044) -> (x*y=w5065:dbl)
                n3197 = To Double Precision Float(number=w5037) -> (double precision float=w5043:dbl)
                n3198 = Build Array(w5043, w5042, w5042, w5042, w5042) -> (w5040:dbl[])
                n3199 = local read "N sets should be saved"() -> (w5046:dbl)
                n3200 = Build Array(w5059, w5054, w5052, w5050, w5048) -> (w5056:dbl[])
                n3201 = Build Array(w5039, w5044, w5065, w5064, w5063, 2.0 ("t")) -> (w5058:dbl[])
                n3202 = Round Toward +Infinity(x=w5046) -> (ceil(x): smallest int >= x=w5047:dbl)
                n3203 = Build Array (concatenate)(w5058, w5057, w5040, w5056) -> (w5055:dbl[])
                n3204 = To Unsigned Long Integer(number=w5047) -> (unsigned 32bit integer=w5045:u32)
              }
              frame 8 {
                w5075 = 0.0 ("f")
                # "MCL raster scan"
                n3205 = local read "Number of scans (MCL)"() -> (w5070:u64)
                n3206 = local read "Scan lines (y)"() -> (w5069:u64)
                n3207 = local read "2D or 1D Scan"() -> (w5072:bool)
                n3208 = local read "Scan Range (V)\n(of steps)"() -> (w5091:dbl)
                n3209 = local read "Fast Scan Dir"() -> (w5098:bool)
                n3210 = local read "Cycles/step (MCL)"() -> (w5088:u64)
                n3211 = local read "Scan steps (MCL)"() -> (w5090:u64)
                n3212 = Select(t=w5069, s=w5072, f=w5070) -> (s? t:f=w5071:u64)
                n3213 = Boolean To (0,1)(Boolean=w5072) -> (0, 1=w5074:i16)
                n3214 = local read "Save ave N"() -> (w5103:dbl)
                n3215 = local read "Initial X"() -> (w5077:dbl)
                n3216 = local read "Initial Y"() -> (w5076:dbl)
                n3217 = To Double Precision Float(number=w5074) -> (double precision float=w5073:dbl)
                n3218 = Boolean To (0,1)(Boolean=w5098) -> (0, 1=w5097:i16)
                n3219 = To Double Precision Float(number=w5071) -> (double precision float=w5086:dbl)
                n3220 = To Double Precision Float(number=w5090) -> (double precision float=w5089:dbl)
                n3221 = To Double Precision Float(number=w5088) -> (double precision float=w5087:dbl)
                n3222 = To Double Precision Float(number=w5097) -> (double precision float=w5096:dbl)
                n3223 = Multiply(x=w5103, y=w5082) -> (x*y=w5102:dbl)
                n3224 = To Double Precision Float(number=w5067) -> (double precision float=w5081:dbl)
                n3225 = local read "N sets should be saved (MCL)"() -> (w5084:dbl)
                n3226 = Build Array(w5081, w5073, w5075, w5075, w5075) -> (w5079:dbl[])
                n3227 = Build Array(w5096, w5091, w5089, w5087, w5086, w5077, w5076) -> (w5093:dbl[])
                n3228 = Build Array(w5078, w5082, w5102, w5101, w5100, 3.0 ("t")) -> (w5095:dbl[])
                n3229 = Round Toward +Infinity(x=w5084) -> (ceil(x): smallest int >= x=w5085:dbl)
                n3230 = Build Array (concatenate)(w5095, w5094, w5079, w5093) -> (w5092:dbl[])
                n3231 = To Unsigned Long Integer(number=w5085) -> (unsigned 32bit integer=w5083:u32)
              }
            }
            n3232 = local read "Index"() -> (w4938:dbl)
            n3233 = call "Create new save file.vi"("Insert"="", "Ext"=".dat", "Index In"=w4938) -> ("Path Out"=w4897:path, "Index Out"=w4910:dbl)
            n3234 = local write "Save file name"(w4897) -> ()
            n3235 = local write "Index"(w4910) -> ()
            n3236 = local write "Save index"(w4910) -> ()
            n3237 = Array Size(array=w4921) -> (size(s)=w4922:i32)
            n3238 = Open/Create/Replace File(file path (use dialog)=w4897, operation (0:open)=T26."create", access (0:read/write)=enum16{"read/write", "read-only", "write-only"}."write-only") -> (refnum out=w4935:refnum<file>)  [unwired: 1 in, 4 out]
            n3239 = local write "Saving..."(TRUE ("Saving...")) -> ()
            n3240 = To Double Precision Float(number=w4922) -> (double precision float=w4920:dbl)
            n3241 = String Length(string="Comment (data description)") -> (length=w4918:i32)
            n3242 = To Double Precision Float(number=w4918) -> (double precision float=w4917:dbl)
            n3243 = Deny Access(7:w4935) -> (3:w4934:refnum<file>)  [unwired: 1 in, 2 out]
            n3244 = Build Array (concatenate)(w4920, w4921, w4917) -> (w4919:dbl[])
            n3245 = case "If fluorescence data to be saved" shown="True" w4908 {
              tunnel: w4897 -> [_ w4987]
              tunnel: [refnum<k0> refnum w4967] -> w4909
              frame False {
              }
              frame True {
                w4966 = 0.0
                n3246 = local read "APD Integration Time (s)"() -> (w4972:dbl)
                n3247 = local read "N APD Samp/step"() -> (w4965:dbl)
                n3248 = Path To String(path=w4987) -> (string=w4986:string)
                n3249 = String Length(string=w4986) -> (length=w4985:i32)
                n3250 = Subtract(x=w4985, y=4) -> (x-y=w4983:i32)
                n3251 = String Subset(string=w4986, length (rest)=w4983) -> (substring=w4982:string)  [unwired: 1 out]
                n3252 = Build Array(w4972, w4965, w4966, w4966, w4966, w4966, w4966, w4966) -> (w4969:dbl[])
                n3253 = Concatenate Strings(w4982, "_fl.dat" ("string")) -> (w4980:string)
                n3254 = Array Size(array=w4969) -> (size(s)=w4971:i32)
                n3255 = String To Path(string=w4980) -> (path=w4976:path)
                n3256 = Open/Create/Replace File(file path (use dialog)=w4976, operation (0:open)=T26."create", access (0:read/write)=enum16{"read/write", "read-only", "write-only"}."write-only") -> (refnum out=w4977:refnum<file>)  [unwired: 1 in, 4 out]
                n3257 = Deny Access(7:w4977) -> (3:w4973:refnum<file>)  [unwired: 1 in, 2 out]
                n3258 = To Double Precision Float(number=w4971) -> (double precision float=w4970:dbl)
                n3259 = Build Array (concatenate)(w4970, w4969) -> (w4968:dbl[])
                n3260 = Write to Binary File(file (use dialog)=w4973, data=w4968, 5:FALSE ("prepend array or string size? (T)"), 9:T25."big-endian, network order" ("byte order (0:big-endian, network order)")) -> (refnum out=w4967:refnum<file>)  [unwired: 1 in, 3 out]
              }
            }
            n3261 = case shown="True" w4895 {
              tunnel: w4897 -> [_ w4949]
              tunnel: [refnum<k0> refnum w4948] -> w4896
              frame False {
              }
              frame True {
                w4944 = 0.0 ("element")
                n3262 = Path To String(path=w4949) -> (string=w4963:string)
                n3263 = Build Array(w4944, w4944, w4944, w4944, w4944, w4944, w4944, w4944) -> (w4945:dbl[])
                n3264 = String Length(string=w4963) -> (length=w4962:i32)
                n3265 = Subtract(x=w4962, y=4) -> (x-y=w4960:i32)
                n3266 = Array Size(array=w4945) -> (size(s)=w4947:i32)
                n3267 = String Subset(string=w4963, length (rest)=w4960) -> (substring=w4959:string)  [unwired: 1 out]
                n3268 = To Double Precision Float(number=w4947) -> (double precision float=w4946:dbl)
                n3269 = Concatenate Strings(w4959, "_pos.dat" ("string")) -> (w4957:string)
                n3270 = Build Array (concatenate)(w4946, w4945) -> (w4943:dbl[])
                n3271 = String To Path(string=w4957) -> (path=w4953:path)
                n3272 = Open/Create/Replace File(file path (use dialog)=w4953, operation (0:open)=T26."create", access (0:read/write)=enum16{"read/write", "read-only", "write-only"}."write-only") -> (refnum out=w4954:refnum<file>)  [unwired: 1 in, 4 out]
                n3273 = Deny Access(7:w4954) -> (3:w4950:refnum<file>)  [unwired: 1 in, 2 out]
                n3274 = Write to Binary File(file (use dialog)=w4950, data=w4943, 5:FALSE ("prepend array or string size? (T)"), 9:T25."big-endian, network order" ("byte order (0:big-endian, network order)")) -> (refnum out=w4948:refnum<file>)  [unwired: 1 in, 3 out]
              }
            }
            n3275 = Write to Binary File(file (use dialog)=w4934, data=w4919, 5:w4915, 9:w4913) -> (refnum out=w4916:refnum<file>)  [unwired: 1 in, 3 out]
            n3276 = Write to Binary File(file (use dialog)=w4916, data="Comment (data description)", 5:w4915, 9:w4913) -> (refnum out=w4912:refnum<file>)  [unwired: 1 in, 3 out]
          }
        }
        n3277 = feedback-in #32(w4856) -> ()
        n3278 = feedback-in #33(w4882) -> ()
        n3279 = feedback-in #34(w4855) -> ()
        n3280 = feedback-in #35(w4866) -> ()
        n3281 = feedback-in #36(w4869) -> ()
        n3282 = feedback-in #37(w4881) -> ()
        n3283 = feedback-in #38(w4872) -> ()
      }
      frame #1 {
        n3284 = local read "Saving..."() -> (w5117:bool)
        n3285 = case shown="True" w5117 {
          tunnel: w5121 -> [_ w5133]
          tunnel: w5120 -> [_ w5146]
          tunnel: w5119 -> [_ w5142]
          tunnel: w5118 -> [_ w5141]
          tunnel: w5116 -> [_ w5122]
          tunnel: w5115 -> [_ w5136]
          tunnel: w5114 -> [_ w5135]
          tunnel: w5113 -> [_ w5134]
          tunnel: w5112 -> [_ w5132]
          tunnel: w5111 -> [_ w5130]
          tunnel: w5110 -> [_ w5129]
          tunnel: w5109 -> [_ w5128]
          tunnel: w5108 -> [_ w5127]
          tunnel: w5107 -> [_ w5126]
          tunnel: w5106 -> [_ w5125]
          tunnel: w5105 -> [_ w5124]
          tunnel: w5104 -> [_ w5123]
          frame False {
          }
          frame True {
            n3286 = Multiply(x=w5133, y=w5132) -> (x*y=→"Time (s)":dbl)
            n3287 = Less Or Equal?(x=w5133, y=w5122) -> (x <= y?=w5144:bool)
            n3288 = Or(x="Stop Saving", y="Abort save 2") -> (x .or. y?=w5137:bool)
            n3289 = Not(x=w5137) -> (.not. x?=w5145:bool)
            n3290 = And(x=w5144, y=w5145) -> (x .and. y?=w5143:bool)
            n3291 = case shown="True" w5143 {
              tunnel: w5146 -> [w5154 w5229]
              tunnel: [0.0 w5232] -> w5140
              tunnel: w5133 -> [_ w5230]
              tunnel: w5122 -> [_ w5231]
              tunnel: w5142 -> [_ w5226]
              tunnel: w5141 -> [_ _]
              tunnel: w5136 -> [w5152 w5219]
              tunnel: w5135 -> [w5151 w5220]
              tunnel: w5134 -> [_ w5218]
              tunnel: w5130 -> [_ w5217]
              tunnel: w5129 -> [_ w5161]
              tunnel: w5128 -> [_ w5210]
              tunnel: w5127 -> [_ w5188]
              tunnel: w5126 -> [w5148 w5170]
              tunnel: w5125 -> [w5149 w5169]
              tunnel: w5124 -> [_ w5166]
              tunnel: w5123 -> [_ w5164]
              frame False {
                w5150 = FALSE
                n3292 = Close File(refnum=w5154) -> ()  [unwired: 1 in, 2 out]
                n3293 = case shown="True" w5151 {
                  tunnel: w5152 -> [_ w5156]
                  frame False {
                  }
                  frame True {
                    n3294 = Close File(refnum=w5156) -> ()  [unwired: 1 in, 2 out]
                  }
                }
                n3295 = case shown="True" w5148 {
                  tunnel: w5149 -> [_ w5155]
                  frame False {
                  }
                  frame True {
                    n3296 = Close File(refnum=w5155) -> ()  [unwired: 1 in, 2 out]
                  }
                }
                n3297 = call <vilib>:"Beep.vi"() -> ()  [unwired: 3 in, 9 out]
                n3298 = local write "Raster Scanning..."(w5150) -> ()
                n3299 = local write "Calibrating..."(w5150) -> ()
                n3300 = property on="Abort wiggle" class="Bool (strict)"("Val(Sgnl)"=TRUE) -> ()  [unwired: 2 in, 2 out]
                n3301 = local write "Stop Saving"(w5150) -> ()
                "Saving..." <- w5150
              }
              frame True {
                n3302 = local read "Calibrating..."() -> (w5221:bool)
                n3303 = case "Write fl. data" shown="True" w5220 {
                  tunnel: w5219 -> [_ w5255]
                  tunnel: w5218 -> [_ w5254]
                  frame False {
                  }
                  frame True {
                    n3304 = Write to Binary File(file (use dialog)=w5255, data=w5254, 5:FALSE ("prepend array or string size? (T)"), 9:T25."big-endian, network order" ("byte order (0:big-endian, network order)")) -> ()  [unwired: 1 in, 4 out]
                  }
                }
                n3305 = Greater?(x="Save ave N", y=1.0) -> (0:w5224:bool)
                n3306 = Not(x=w5221) -> (.not. x?=w5223:bool)
                n3307 = And(x=w5223, y=w5224) -> (x .and. y?=w5167:bool)
                n3308 = case shown="True" w5167 {
                  tunnel: w5166 -> [w5235 w5246]
                  tunnel: [w5235 w5238] -> w5165
                  tunnel: "Save ave N" -> [_ w5239]
                  frame False {
                  }
                  frame True {
                    w5236 = 2 ("dimension size")
                    n3309 = Array Size(array=w5246) -> (size(s)=w5240:i32)
                    n3310 = Divide(x=w5240, y=w5236) -> (x/y=w5244:dbl)
                    n3311 = Reshape Array(w5246, w5244, w5236) -> (w5245:u64[][])
                    n3312 = Transpose 2D Array(2D array=w5245) -> (transposed array=w5243:u64[][])
                    n3313 = for {
                      tunnel: w5243 -> [w5248] mode=indexing
                      tunnel: [w5247] -> w5237 mode=indexing
                      tunnel: w5239 -> [w5249]
                      workers-P: _ -> [_]
                      n3314 = call "downsample 1D array - U64.vi"("Ave N"=w5249, "Array In"=w5248) -> ("Array Out"=w5247:u64[])  [unwired: 1 in]
                    }
                    n3315 = Transpose 2D Array(2D array=w5237) -> (transposed array=w5242:u64[][])
                    n3316 = Divide(x=w5240, y=w5239) -> (x/y=w5241:dbl)
                    n3317 = Reshape Array(w5242, w5241) -> (w5238:u64[])
